vi "Write SPI Configuration.vi"(8 "error in (no error)":errorcluster, 10 "SPI Configuration":T1, 11 "Bus Configuration.lvclass":refnum<class "Bus Configuration.lvclass">) -> (0 "error out":errorcluster, 3 "Bus Configuration.lvclass":refnum<class "Bus Configuration.lvclass">)   [LabVIEW 2014, in "Bus Configuration.lvclass"]
uses:
  Bus Configuration/Bus Configuration.lvclass
  SPI Configuration.ctl
  <vilib>/NI/Configuration Framework/serializable configuration/NISE_CEF_serializable configuration.lvclass
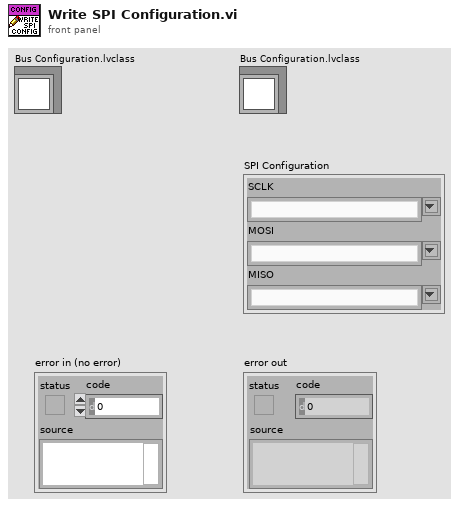
[diagram p1: front panel]
types:
  T1 = typedef "Bus Configuration.lvclass/SPI Configuration.ctl" = cluster{"SCLK":string, "MOSI":string, "MISO":string}
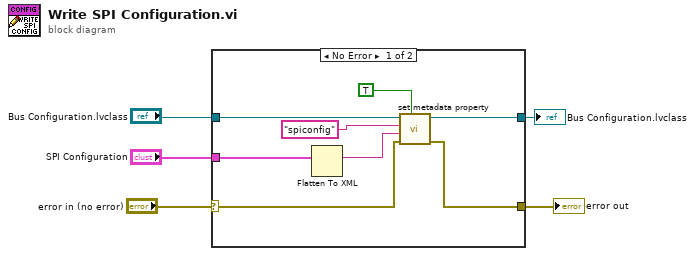
[diagram p0: block diagram]
diagram:
  n1 = case shown="No Error" "error in (no error)" {
    selector: "error in (no error)" -> [w9 w15]
    tunnel: "SPI Configuration" -> [w7 _]
    tunnel: "Bus Configuration.lvclass" -> [w13 w14]
    tunnel: [w6 w14] -> w1
    tunnel: [w11 w15] -> w4
    frame No Error {
      n2 = Flatten To XML(anything=w7) -> (xml string=w10:string)
      n3 = call <vilib>:"set metadata property.vi"("overwrite?"=TRUE, "error in"=w9, "value"=w10, "key"="spiconfig", "configuration in"=w13) -> ("error out"=w11:errorcluster, "configuration out"=w6:refnum<class "Bus Configuration.lvclass">)  [unwired: 5 in]
    }
    frame Error {
    }
  }
  "error out" <- w4
  "Bus Configuration.lvclass" <- w1
